vi "PAN_SchedulerMgr.vi"(8 "error in (no error)":errorcluster, 10 "action":T2, 11 "command":string) -> (0 "error out":errorcluster, 2 "execute now":T1[](array[typedef]))   [LabVIEW 2016]
uses:
  PAN_Scheduler_action.ctl
  PAN_scheduler_element.ctl
panel:
  out "schedule":T1[](array[typedef])
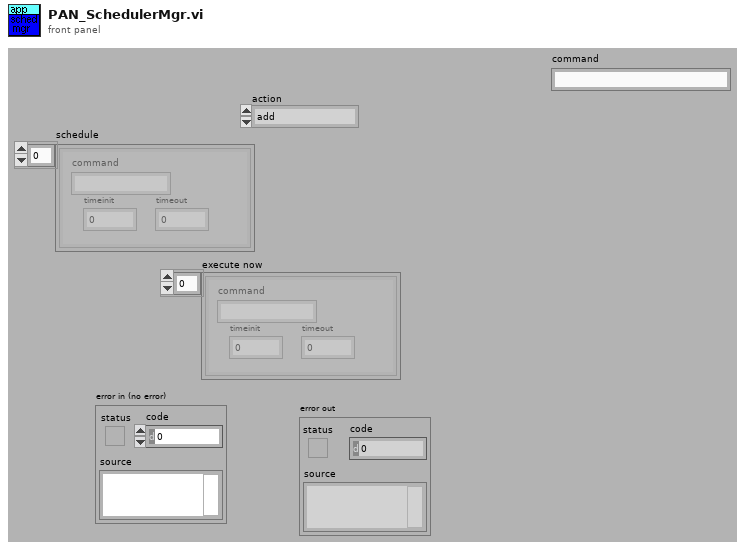
[diagram p1: front panel]
types:
  T1 = typedef "PAN_scheduler_element.ctl" = cluster{"command":string, "timeinit":i32, "timeout":i32}
  T2 = typedef "PAN_Scheduler_action.ctl" = enum16{"add", "search", "clean", "get all"}
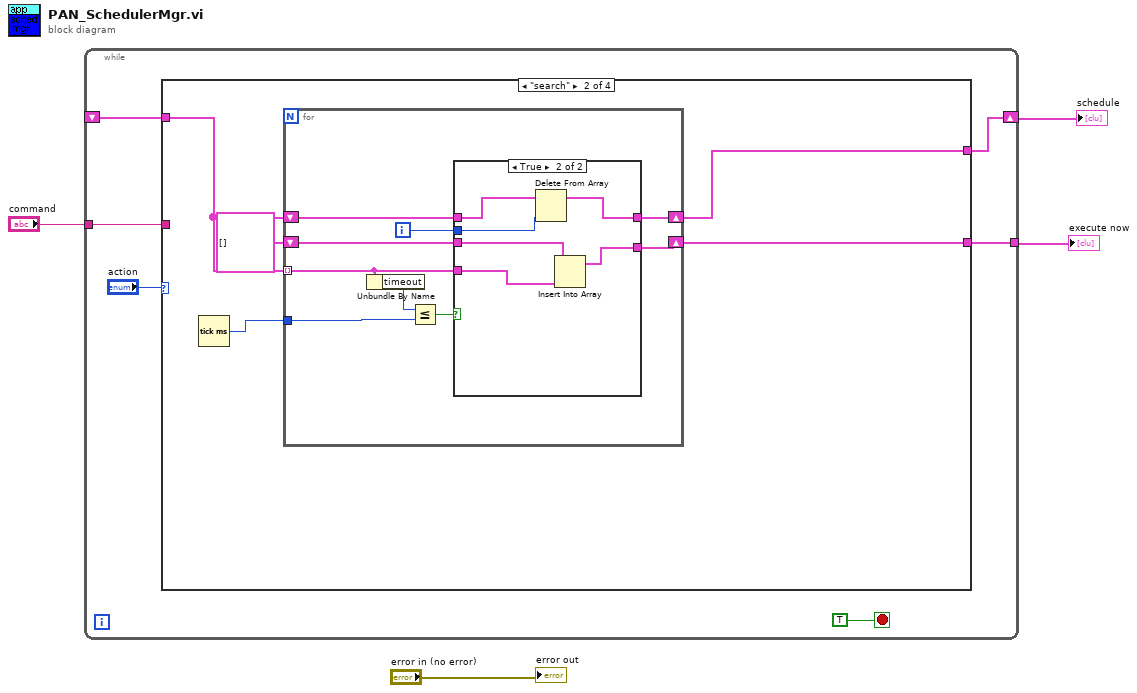
[diagram p0: block diagram]
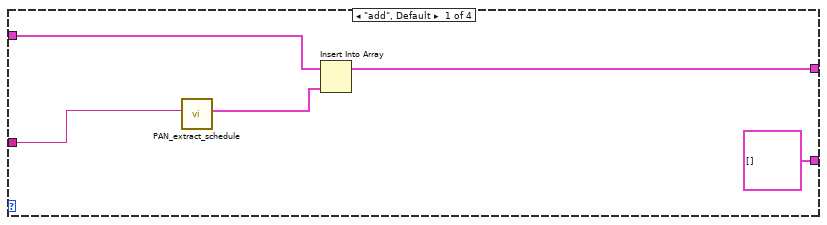
[diagram p2: hidden frame]
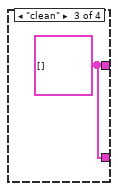
[diagram p4: hidden frame]
diagram:
  n1 = while {
    shift-right: [w5] -> w1
    shift-left: _ -> [w6]
    tunnel: [w8] -> w4
    tunnel: "command" -> [w7]
    stop <- TRUE stop-if-true
    n2 = case shown="\"search\"" "action" {
      tunnel: w6 -> [w15 w19 _ w39]
      tunnel: [T1[] [] w17 w38 w39] -> w8
      tunnel: w7 -> [w13 _ _ _]
      tunnel: [w14 w18 w38 w39] -> w5
      frame "add", Default {
        n3 = call "PAN_extract_schedule.vi"("command"=w13) -> ("schedule"=w12:T1[])  [unwired: 10 out]
        n4 = Insert Into Array(array=w15, new element=w12) -> (w14:T1[])  [unwired: 1 in]
      }
      frame "search" {
        n5 = Tick Count (ms)() -> (millisecond timer value=w20:u32)
        n6 = for {
          tunnel: w19 -> [w26] mode=indexing
          tunnel: w20 -> [w28]
          shift-right: [w25] -> w17
          shift-left: T1[] [] -> [w21]
          shift-right: [w22] -> w18
          shift-left: w19 -> [w24]
          i -> [w23]
          n7 = Unbundle By Name(w26) -> ("timeout"=w29:i32)
          n8 = Less Or Equal?(x=w29, y=w28) -> (x <= y?=w27:bool)
          n9 = case shown="True" w27 {
            tunnel: w26 -> [_ w34]
            tunnel: [w30 w33] -> w25
            tunnel: w24 -> [w31 w37]
            tunnel: w23 -> [_ w36]
            tunnel: [w31 w35] -> w22
            tunnel: w21 -> [w30 w32]
            frame False {
            }
            frame True {
              n10 = Delete From Array(array=w37, index=w36) -> (array with subset deleted=w35:T1[])  [unwired: 1 in, 1 out]
              n11 = Insert Into Array(array=w32, new element=w34) -> (w33:T1[])  [unwired: 1 in]
            }
          }
        }
      }
      frame "clean" {
        w38 = T1[] []
      }
      frame "get all" {
      }
    }
  }
  "schedule" <- w1
  "execute now" <- w4
  "error out" <- "error in (no error)"
